vi "Read Compressed Image (FPGA) (SubVI).vi"() -> (0 "Output Valid":bool, 3 "Data Out":u8)   [LabVIEW 2014]
uses:
  Uncompression States.ctl
  <vilib>/rvi/interface/RandomDataEmulation/niFpgaRandomDataHandleErrors.vi
  <vilib>/rvi/DataTransferAndStorage/Container/XNode/niFpgaContainer.xnode
  <vilib>/rvi/interface/RandomDataEmulation/nirviRandomDataFpgaReadWriteTemplate.vi
  <vilib>/rvi/FXPMathLib/FxpMul/XNode/nifxpmath_Multiplier.xnode
  <vilib>/rvi/FXPMathLib/sim/FxpSim.dll
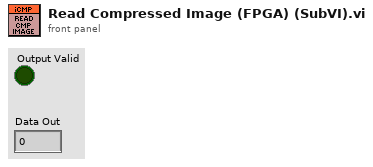
[diagram p1: front panel]
types:
  T1 = typedef "Uncompression States.ctl" = enum16{"Read BD-MIN", "Read IMG DATA", "Send Block Data"}
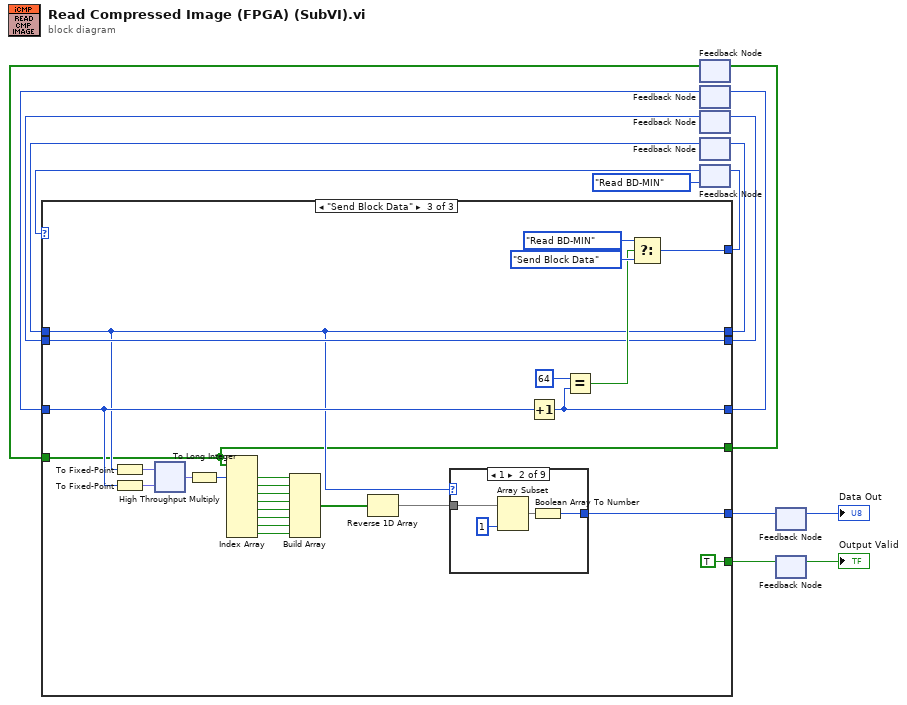
[diagram p0: block diagram]
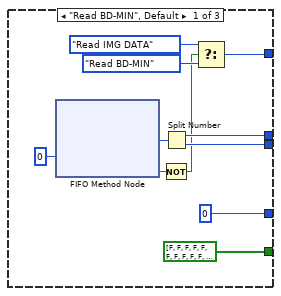
[diagram p2: hidden frame]
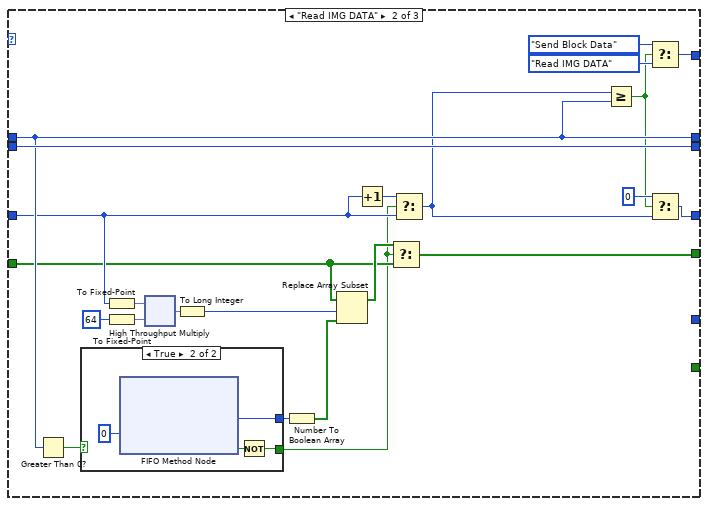
[diagram p3: hidden frame]
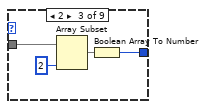
[diagram p6: hidden frame]
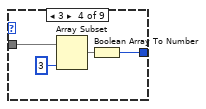
[diagram p7: hidden frame]
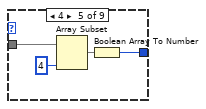
[diagram p8: hidden frame]
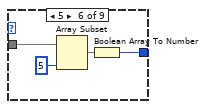
[diagram p9: hidden frame]
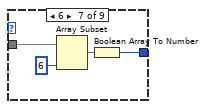
[diagram p10: hidden frame]
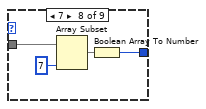
[diagram p11: hidden frame]
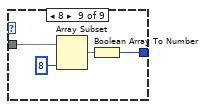
[diagram p12: hidden frame]
diagram:
  n1 = feedback #1() -> (w8:bool[])  [unwired: 1 in]
  n2 = feedback #2() -> (w10:u8)  [unwired: 1 in]
  n3 = feedback #3() -> (w7:u8)  [unwired: 1 in]
  n4 = feedback #4() -> (w6:u8)  [unwired: 1 in]
  n5 = feedback #5(Uncompression_States."Read BD-MIN") -> (w4:T1)
  n6 = case shown="\"Send Block Data\"" w4 {
    tunnel: [w20 w43 w75] -> w3
    tunnel: [w22 w46 w69] -> w11
    tunnel: [w21 w49 w72] -> w12
    tunnel: w6 -> [_ w46 w69]
    tunnel: w7 -> [_ w49 w72]
    tunnel: [bool[] [FALSE, FALSE, FALSE, FALSE, FALSE, FALSE, FALSE, FALSE, FALSE, FALSE, FALSE, FALSE, FALSE, FALSE, FALSE, FALSE, FALSE, FALSE, FALSE, FALSE, FALSE, FALSE, FALSE, FALSE, FALSE, FALSE, FALSE, FALSE, FALSE, FALSE, FALSE, FALSE, FALSE, FALSE, FALSE, FALSE, FALSE, FALSE, FALSE, FALSE, FALSE, FALSE, FALSE, FALSE, FALSE, FALSE, FALSE, FALSE, FALSE, FALSE, FALSE, FALSE, FALSE, FALSE, FALSE, FALSE, FALSE, FALSE, FALSE, FALSE, FALSE, FALSE, FALSE, FALSE, FALSE, FALSE, FALSE, FALSE, FALSE, FALSE, FALSE, FALSE, FALSE, FALSE, FALSE, FALSE, FALSE, FALSE, FALSE, FALSE, FALSE, FALSE, FALSE, FALSE, FALSE, FALSE, FALSE, FALSE, FALSE, FALSE, FALSE, FALSE, FALSE, FALSE, FALSE, FALSE, FALSE, FALSE, FALSE, FALSE, FALSE, FALSE, FALSE, FALSE, FALSE, FALSE, FALSE, FALSE, FALSE, FALSE, FALSE, FALSE, FALSE, FALSE, FALSE, FALSE, FALSE, FALSE, FALSE, FALSE, FALSE, FALSE, FALSE, FALSE, FALSE, FALSE, FALSE, FALSE, FALSE, FALSE, FALSE, FALSE, FALSE, FALSE, FALSE, FALSE, FALSE, FALSE, FALSE, FALSE, FALSE, FALSE, FALSE, FALSE, FALSE, FALSE, FALSE, FALSE, FALSE, FALSE, FALSE, FALSE, FALSE, FALSE, FALSE, FALSE, FALSE, FALSE, FALSE, FALSE, FALSE, FALSE, FALSE, FALSE, FALSE, FALSE, FALSE, FALSE, FALSE, FALSE, FALSE, FALSE, FALSE, FALSE, FALSE, FALSE, FALSE, FALSE, FALSE, FALSE, FALSE, FALSE, FALSE, FALSE, FALSE, FALSE, FALSE, FALSE, FALSE, FALSE, FALSE, FALSE, FALSE, FALSE, FALSE, FALSE, FALSE, FALSE, FALSE, FALSE, FALSE, FALSE, FALSE, FALSE, FALSE, FALSE, FALSE, FALSE, FALSE, FALSE, FALSE, FALSE, FALSE, FALSE, FALSE, FALSE, FALSE, FALSE, FALSE, FALSE, FALSE, FALSE, FALSE, FALSE, FALSE, FALSE, FALSE, FALSE, FALSE, FALSE, FALSE, FALSE, FALSE, FALSE, FALSE, FALSE, FALSE, FALSE, FALSE, FALSE, FALSE, FALSE, FALSE, FALSE, FALSE, FALSE, FALSE, FALSE, FALSE, FALSE, FALSE, FALSE, FALSE, FALSE, FALSE, FALSE, FALSE, FALSE, FALSE, FALSE, FALSE, FALSE, FALSE, FALSE, FALSE, FALSE, FALSE, FALSE, FALSE, FALSE, FALSE, FALSE, FALSE, FALSE, FALSE, FALSE, FALSE, FALSE, FALSE, FALSE, FALSE, FALSE, FALSE, FALSE, FALSE, FALSE, FALSE, FALSE, FALSE, FALSE, FALSE, FALSE, FALSE, FALSE, FALSE, FALSE, FALSE, FALSE, FALSE, FALSE, FALSE, FALSE, FALSE, FALSE, FALSE, FALSE, FALSE, FALSE, FALSE, FALSE, FALSE, FALSE, FALSE, FALSE, FALSE, FALSE, FALSE, FALSE, FALSE, FALSE, FALSE, FALSE, FALSE, FALSE, FALSE, FALSE, FALSE, FALSE, FALSE, FALSE, FALSE, FALSE, FALSE, FALSE, FALSE, FALSE, FALSE, FALSE, FALSE, FALSE, FALSE, FALSE, FALSE, FALSE, FALSE, FALSE, FALSE, FALSE, FALSE, FALSE, FALSE, FALSE, FALSE, FALSE, FALSE, FALSE, FALSE, FALSE, FALSE, FALSE, FALSE, FALSE, FALSE, FALSE, FALSE, FALSE, FALSE, FALSE, FALSE, FALSE, FALSE, FALSE, FALSE, FALSE, FALSE, FALSE, FALSE, FALSE, FALSE, FALSE, FALSE, FALSE, FALSE, FALSE, FALSE, FALSE, FALSE, FALSE, FALSE, FALSE, FALSE, FALSE, FALSE, FALSE, FALSE, FALSE, FALSE, FALSE, FALSE, FALSE, FALSE, FALSE, FALSE, FALSE, FALSE, FALSE, FALSE, FALSE, FALSE, FALSE, FALSE, FALSE, FALSE, FALSE, FALSE, FALSE, FALSE, FALSE, FALSE, FALSE, FALSE, FALSE, FALSE, FALSE, FALSE, FALSE, FALSE, FALSE, FALSE, FALSE, FALSE, FALSE, FALSE, FALSE, FALSE, FALSE, FALSE, FALSE, FALSE, FALSE, FALSE, FALSE, FALSE, FALSE, FALSE, FALSE, FALSE, FALSE, FALSE, FALSE, FALSE, FALSE, FALSE, FALSE, FALSE, FALSE, FALSE, FALSE, FALSE, FALSE, FALSE, FALSE, FALSE, FALSE, FALSE, FALSE, FALSE, FALSE, FALSE, FALSE, FALSE, FALSE, FALSE, FALSE, FALSE, FALSE, FALSE, FALSE, FALSE, FALSE, FALSE, FALSE, FALSE, FALSE, FALSE, FALSE, FALSE, FALSE, FALSE, FALSE, FALSE, FALSE, FALSE, FALSE, FALSE, FALSE, FALSE, FALSE, FALSE, FALSE, FALSE, FALSE, FALSE, FALSE, FALSE, FALSE, FALSE, FALSE, FALSE, FALSE, FALSE, FALSE] ("initialized array") w35 w58] -> w13
    tunnel: w8 -> [_ w33 w58]
    tunnel: [u8 0 ("Timeout") w32 w79] -> w9
    tunnel: w10 -> [_ w41 w71]
    tunnel: [_ _ TRUE] -> w15
    tunnel: [_ _ w59] -> w14
    frame "Read BD-MIN", Default {
      n7 = xnode ("FIFO Method Node")("Timeout"=0) -> ("Element"=w25:u16, "Timed Out?"=w24:bool)  [unwired: 1 in, 1 out]
      n8 = Not(x=w24) -> (.not. x?=w18:bool)
      n9 = Split Number(x=w25) -> (hi(x)=w22:u8, lo(x)=w21:u8)
      n10 = Select(t=Uncompression_States."Read IMG DATA", s=w18, f=Uncompression_States."Read BD-MIN") -> (s? t:f=w20:T1)
    }
    frame "Read IMG DATA" {
      n11 = Greater Than 0?(x=w46) -> (x > 0?=w48:bool)
      n12 = case shown="True" w48 {
        tunnel: [_ w51] -> w31
        tunnel: [_ w50] -> w37
        frame False {
        }
        frame True {
          n13 = xnode ("FIFO Method Node")("Timeout"=0) -> ("Element"=w50:u64, "Timed Out?"=w52:bool)  [unwired: 1 in, 1 out]
          n14 = Not(x=w52) -> (.not. x?=w51:bool)
        }
      }
      n15 = To Fixed-Point(number=w41) -> (fixed-point=w28:fxp<+,8,8>)  [unwired: 1 in]
      n16 = To Fixed-Point(number=u8 64 ("y")) -> (fixed-point=w27:fxp<+,8,8>)  [unwired: 1 in]
      n17 = xnode "High Throughput Multiply"("x"=w28, "y"=w27) -> ("x*y"=w39:fxp<+,9,9>)
      n18 = To Long Integer(number=w39) -> (32bit integer=w38:i32)
      n19 = Number To Boolean Array(number=w37) -> (Boolean array=w36:bool[])
      n20 = Replace Array Subset(array=w33, new element=w36, index=w38) -> (w34:bool[])
      n21 = Increment(x=w41) -> (x+1=w47:u8)
      n22 = Select(t=w34, s=w31, f=w33) -> (s? t:f=w35:bool[])
      n23 = Select(t=w47, s=w31, f=w41) -> (s? t:f=w42:u8)
      n24 = Greater Or Equal?(x=w42, y=w46) -> (x >= y?=w29:bool)
      n25 = Select(t=Uncompression_States."Send Block Data", s=w29, f=Uncompression_States."Read IMG DATA") -> (s? t:f=w43:T1)
      n26 = Select(t=u8 0, s=w29, f=w42) -> (s? t:f=w32:u8)
    }
    frame "Send Block Data" {
      n27 = To Fixed-Point(number=w69) -> (fixed-point=w55:fxp<+,8,8>)  [unwired: 1 in]
      n28 = To Fixed-Point(number=w71) -> (fixed-point=w56:fxp<+,8,8>)  [unwired: 1 in]
      n29 = xnode ("High Throughput Multiply")("x"=w55, "y"=w56) -> ("x*y"=w70:fxp<+,9,9>)
      n30 = To Long Integer(number=w70) -> (32bit integer=w57:i32)
      n31 = Index Array(array=w58, index #1=w57) -> (element #1=w68:bool, element #2=w67:bool, element #3=w66:bool, element #4=w65:bool, element #5=w64:bool, element #6=w63:bool, element #7=w62:bool, element #8=w61:bool)  [unwired: 7 in]
      n32 = Build Array(w68, w67, w66, w65, w64, w63, w62, w61) -> (w60:bool[])
      n33 = Reverse 1D Array(array=w60) -> (reversed array=w54:bool[])
      n34 = case shown="1" w69 {
        tunnel: w54 -> [_ w83 w87 w91 w95 w99 w103 w107 w111]
        tunnel: [_ w80 w84 w88 w92 w96 w100 w104 w108] -> w59
        frame 0, Default {
        }
        frame 1 {
          n35 = Array Subset(array=w83, length=1) -> (w81:bool[])  [unwired: 1 in]
          n36 = Boolean Array To Number(Boolean array=w81) -> (number=w80:u8)
        }
        frame 2 {
          n37 = Array Subset(array=w87, length=2) -> (w85:bool[])  [unwired: 1 in]
          n38 = Boolean Array To Number(Boolean array=w85) -> (number=w84:u8)
        }
        frame 3 {
          n39 = Array Subset(array=w91, length=3) -> (w89:bool[])  [unwired: 1 in]
          n40 = Boolean Array To Number(Boolean array=w89) -> (number=w88:u8)
        }
        frame 4 {
          n41 = Array Subset(array=w95, length=4) -> (w93:bool[])  [unwired: 1 in]
          n42 = Boolean Array To Number(Boolean array=w93) -> (number=w92:u8)
        }
        frame 5 {
          n43 = Array Subset(array=w99, length=5) -> (w97:bool[])  [unwired: 1 in]
          n44 = Boolean Array To Number(Boolean array=w97) -> (number=w96:u8)
        }
        frame 6 {
          n45 = Array Subset(array=w103, length=6) -> (w101:bool[])  [unwired: 1 in]
          n46 = Boolean Array To Number(Boolean array=w101) -> (number=w100:u8)
        }
        frame 7 {
          n47 = Array Subset(array=w107, length=7) -> (w105:bool[])  [unwired: 1 in]
          n48 = Boolean Array To Number(Boolean array=w105) -> (number=w104:u8)
        }
        frame 8 {
          n49 = Array Subset(array=w111, length=8) -> (w109:bool[])  [unwired: 1 in]
          n50 = Boolean Array To Number(Boolean array=w109) -> (number=w108:u8)
        }
      }
      n51 = Increment(x=w71) -> (x+1=w79:u8)
      n52 = Equal?(x=u8 64, y=w79) -> (x = y?=w74:bool)
      n53 = Select(t=Uncompression_States."Read BD-MIN", s=w74, f=Uncompression_States."Send Block Data") -> (s? t:f=w75:T1)
    }
  }
  n54 = feedback-in #1(w13) -> ()
  n55 = feedback-in #2(w9) -> ()
  n56 = feedback-in #3(w12) -> ()
  n57 = feedback-in #4(w11) -> ()
  n58 = feedback-in #5(w3) -> ()
  n59 = feedback-in #6(w14) -> ()
  n60 = feedback #6() -> (→"Data Out":u8)  [unwired: 1 in]
  n61 = feedback-in #7(w15) -> ()
  n62 = feedback #7() -> (→"Output Valid":bool)  [unwired: 1 in]
